vi "Insert Images into DB.vi"() -> ()   [LabVIEW 2024]
uses:
  <vilib>/drjdpowell/SQLite Library/SQL Connection/Open (path).vi
  <vilib>/drjdpowell/SQLite Library/SQL Connection/Open (string).vi
  <vilib>/AdvancedString/Path To Command Line String.vi
  <vilib>/drjdpowell/SQLite Library/SQL Connection/Execute SQL (Single Integer).vi
  <vilib>/drjdpowell/SQLite Library/SQL Connection/Execute SQL (No results).vi
  <vilib>/drjdpowell/SQLite Library/SQL Connection/Connection.lvclass
  <vilib>/drjdpowell/SQLite Library/SQLite.lvlib
panel:
  in  "db file":path
  in  "# imgs":i32
  in  "img folder":path
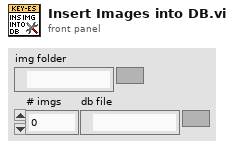
[diagram p1: front panel]
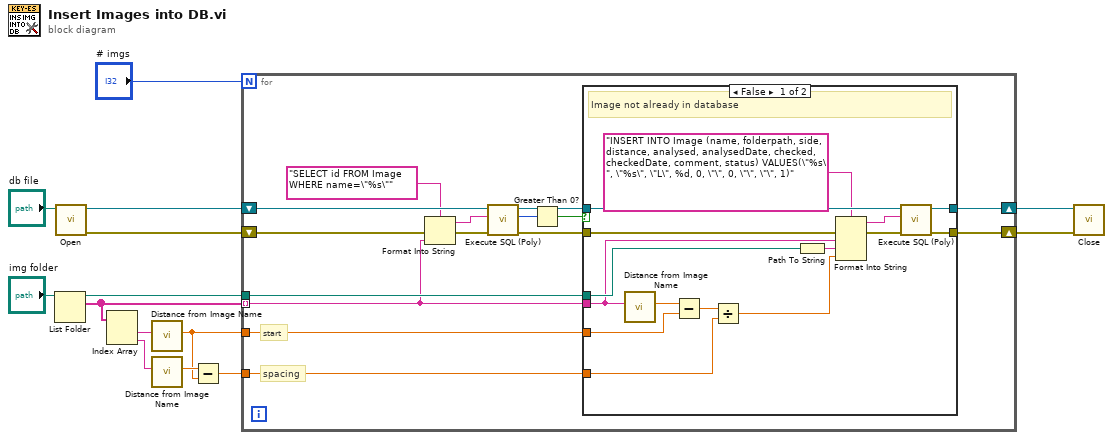
[diagram p0: block diagram]
diagram:
  n1 = List Folder(path="img folder") -> (path out=w8:path, filenames=w6:string[])  [unwired: 3 in, 2 out]
  n2 = call-poly <vilib>:"Open.vi"("db file"="db file") -> ("error out"=w10:errorcluster, "SQLite Connection"=w12:refnum<class "Connection.lvclass">)  [unwired: 9 in]
  n3 = Index Array(array=w6) -> (element #1=w5:string, element #2=w4:string)  [unwired: 2 in]
  n4 = call "Distance from Image Name.vi"("Image Name"=w5) -> ("Distance (km)"=w2:dbl)  [unwired: 10 in]
  n5 = call "Distance from Image Name.vi"("Image Name"=w4) -> ("Distance (km)"=w3:dbl)  [unwired: 10 in]
  n6 = Subtract(x=w3, y=w2) -> (x-y=w1:dbl)
  n7 = for {
    N: "# imgs" -> [_]
    tunnel: w6 -> [w17] mode=indexing
    shift-right: [w27] -> w11
    shift-left: w12 -> [w29]
    shift-right: [w26] -> w9
    shift-left: w10 -> [w24]
    tunnel: w8 -> [w18]
    tunnel: w2 -> [w16]
    tunnel: w1 -> [w15]
    # "spacing"
    # "start"
    n8 = Format Into String(format string="SELECT id FROM Image WHERE name=\"%s\"", error in=w24, w17) -> (resulting string=w22:string, error out=w23:errorcluster)  [unwired: 1 in]
    n9 = call-poly <vilib>:"Execute SQL (Poly).vi"("error in (no error)"=w23, "SQL"=w22, "SQLite Connection in"=w29) -> ("error out"=w20:errorcluster, "Result"=w21:i64, "SQLite Connection"=w28:refnum<class "Connection.lvclass">)  [unwired: 6 in]
    n10 = Greater Than 0?(x=w21) -> (x > 0?=w19:bool)
    n11 = case shown="False" w19 {
      tunnel: w28 -> [w44 w46]
      tunnel: [w43 w46] -> w27
      tunnel: [w42 w45] -> w26
      tunnel: w20 -> [w39 w45]
      tunnel: w18 -> [w36 _]
      tunnel: w17 -> [w35 _]
      tunnel: w16 -> [w33 _]
      tunnel: w15 -> [w31 _]
      frame False {
        # "Image not already in database"
        n12 = call "Distance from Image Name.vi"("Image Name"=w35) -> ("Distance (km)"=w34:dbl)  [unwired: 10 in]
        n13 = Subtract(x=w34, y=w33) -> (x-y=w32:dbl)
        n14 = Divide(x=w32, y=w31) -> (x/y=w30:dbl)
        n15 = Path To String(path=w36) -> (string=w37:string)
        n16 = Format Into String(format string="INSERT INTO Image (name, folderpath, side, distance, analysed, analysedDate, checked, checkedDate, comment, status) VALUES(\"%s\", \"%s\", \"L\", %d, 0, \"\", 0, \"\", \"\", 1)", error in=w39, w35, w37, w30) -> (resulting string=w40:string, error out=w38:errorcluster)  [unwired: 1 in]
        n17 = call-poly <vilib>:"Execute SQL (Poly).vi"("error in (no error)"=w38, "SQL"=w40, "SQLite Connection in"=w44) -> ("error out"=w42:errorcluster, "SQLite Connection"=w43:refnum<class "Connection.lvclass">)  [unwired: 7 in]
      }
      frame True {
        # "Image already in database"
      }
    }
  }
  n18 = call-dynamic "Close.vi"("error in (no error)"=w9, "SQLite Connection in"=w11) -> ()  [unwired: 9 in, 1 out]
